vi "Instantiate.vi"(0 "location":string, 5 "insecurePort":string, 11 "error in (no error)":errorcluster) -> (4 "Measurement Client Wrapper out":refnum<class "Measurement Client Wrapper.lvclass">, 15 "error out":errorcluster)   [LabVIEW 2020, in "Measurement Client Wrapper.lvclass"]
uses:
  Measurement Client Wrapper.lvclass
  Measurement Client Wrapper.lvclass/Measurement Client Wrapper.ctl
  Measurement_lv_client/Measurement_lv_client Class/Measurement_lv_client.lvclass
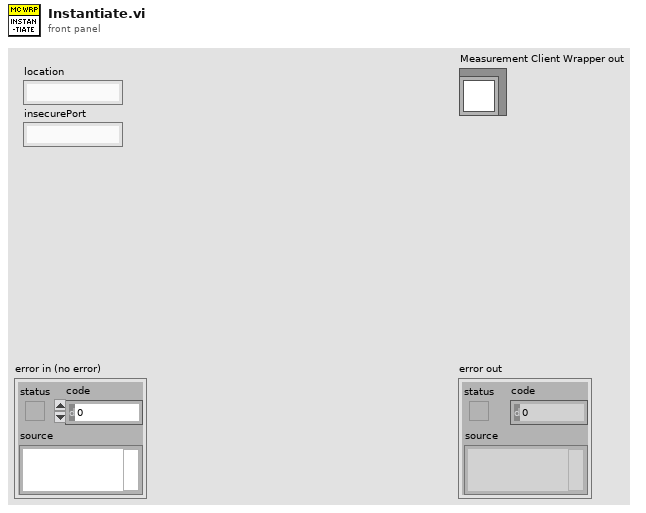
[diagram p1: front panel]
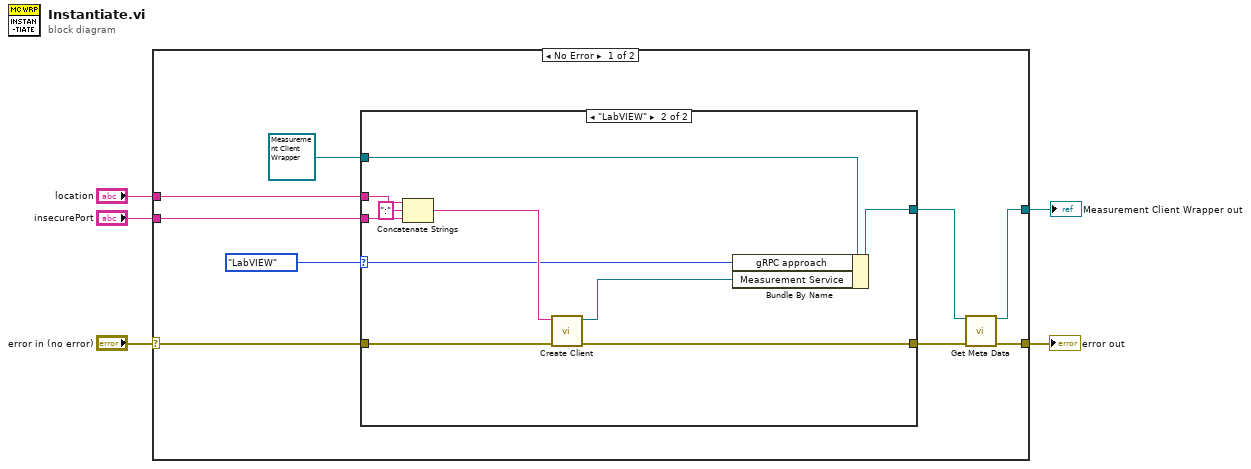
[diagram p0: block diagram]
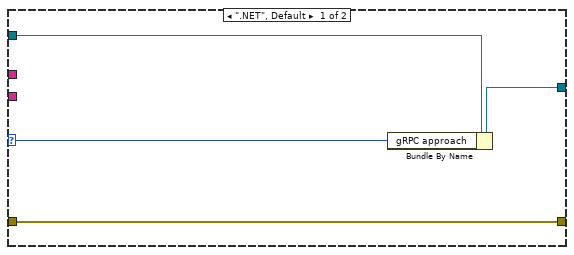
[diagram p2: hidden frame]
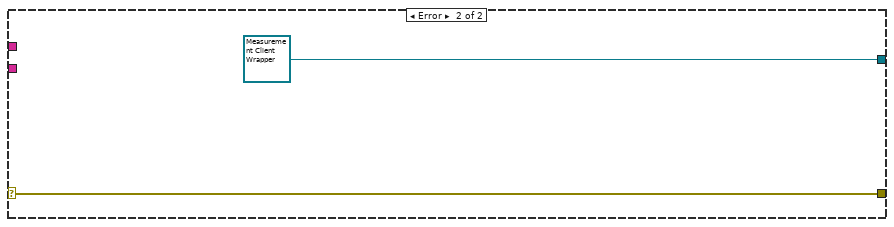
[diagram p3: hidden frame]
diagram:
  n1 = case shown="No Error" "error in (no error)" {
    selector: "error in (no error)" -> [w14 w30]
    tunnel: [w8 w30] -> w4
    tunnel: [w6 refnum<class "Measurement Client Wrapper.lvclass"> refnum ("Measurement Client Wrapper out")] -> w3
    tunnel: "location" -> [w13 _]
    tunnel: "insecurePort" -> [w12 _]
    frame No Error {
      n2 = case shown="\"LabVIEW\"" enum16{".NET", "LabVIEW"}."LabVIEW" ("gRPC approach") {
        selector: enum16{".NET", "LabVIEW"}."LabVIEW" ("gRPC approach") -> [w16 w20]
        tunnel: [w18 w19] -> w7
        tunnel: w14 -> [w17 w28]
        tunnel: [w17 w23] -> w9
        tunnel: w13 -> [_ w27]
        tunnel: w12 -> [_ w26]
        tunnel: refnum<class "Measurement Client Wrapper.lvclass"> refnum ("Measurement Client Wrapper out") -> [w15 w22]
        frame ".NET", Default {
          n3 = Bundle By Name(cluster=w15, "gRPC approach"=w16) -> (w18:refnum<class "Measurement Client Wrapper.lvclass">)
        }
        frame "LabVIEW" {
          n4 = Concatenate Strings(w27, ":" ("string"), w26) -> (w24:string)
          n5 = call "Create Client.vi"("error in (no error)"=w28, "address"=w24) -> ("error out"=w23:errorcluster, "gRPC Client out"=w21:refnum<class "Measurement_lv_client.lvclass">)  [unwired: 8 in]
          n6 = Bundle By Name(cluster=w22, "gRPC approach"=w20, "Measurement Service"=w21) -> (w19:refnum<class "Measurement Client Wrapper.lvclass">)
        }
      }
      n7 = call "Get Meta Data.vi"("Measurement Client Wrapper in"=w7, "error in"=w9) -> ("Measurement Client Wrapper out"=w6:refnum<class "Measurement Client Wrapper.lvclass">, "error out"=w8:errorcluster)  [unwired: 12 in]
    }
    frame Error {
    }
  }
  "error out" <- w4
  "Measurement Client Wrapper out" <- w3
